vi "sedSpectrometer_acceptCommand_stopImageCapture.vi"(8 "error in (no error)":errorcluster, 11 "command_stopImageCapture_Ctl":T1) -> (0 "error out":errorcluster, 2 "function return":i32, 3 "command_stopImageCapture_Ctl out":T1)   [LabVIEW 2016, in "SALLV_sedSpectrometer.lvlib"]
doc: "int sedSpectrometer_shm_acceptCommand_stopImageCaptureLV(sedSpectrometer_command_stopImageCaptureLV *command_stopImageCapture_Ctl );"
uses:
  SALLV_sedSpectrometer.lvlib
  DataTypes/command_stopImageCapture.ctl
  SALLV_sedSpectrometer.so
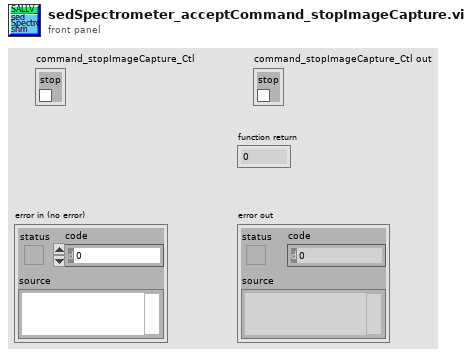
[diagram p1: front panel]
types:
  T1 = typedef "SALLV_sedSpectrometer.lvlib/command_stopImageCapture.ctl" = cluster{"stop":bool}
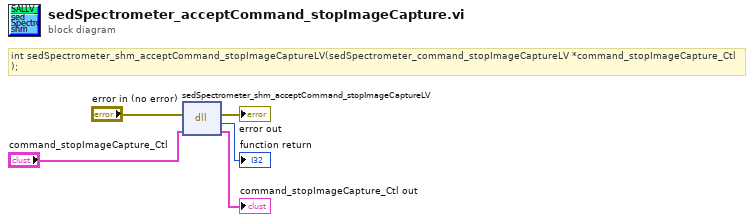
[diagram p0: block diagram]
diagram:
  # "int sedSpectrometer_shm_acceptCommand_stopImageCaptureLV(sedSpectrometer_command_stopImageCaptureLV *command_stopImageCapture_Ctl );"
  n1 = dll-call lib="home/harini/TCS/ts_sallv_sedSpectrometer/SALLV_sedSpectrometer.*" fn="sedSpectrometer_shm_acceptCommand_stopImageCaptureLV"(error in="error in (no error)", "command_stopImageCapture_Ctl"="command_stopImageCapture_Ctl") -> (error out=→"error out":errorcluster, →"function return":i32, "command_stopImageCapture_Ctl"=→"command_stopImageCapture_Ctl out":T1)  [unwired: 2 in, 1 out]
